vi "ComputeRelativeXYJoystickPosition.vi"(5 "Joystick Axis Info":T1, 6 "Joystick Offset":T2, 7 "reference":refnum<vi>) -> (3 "Rel XY Pos":T3)   [LabVIEW 2014]
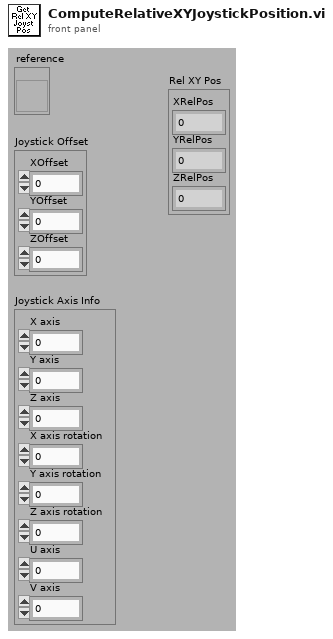
[diagram p1: front panel]
types:
  T1 = cluster{"X axis":i32, "Y axis":i32, "Z axis":i32, "X axis rotation":i32, "Y axis rotation":i32, "Z axis rotation":i32, "U axis":i32, "V axis":i32}
  T2 = cluster{"XOffset":i32, "YOffset":i32, "ZOffset":i32}
  T3 = cluster{"XRelPos":i32, "YRelPos":i32, "ZRelPos":i32}
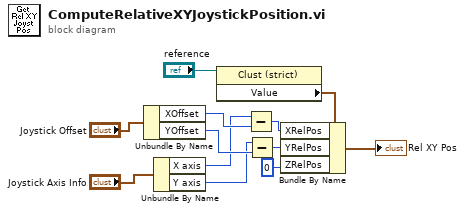
[diagram p0: block diagram]
diagram:
  n1 = Unbundle By Name("Joystick Offset") -> ("XOffset"=w8:i32, "YOffset"=w10:i32)
  n2 = Unbundle By Name("Joystick Axis Info") -> ("X axis"=w7:i32, "Y axis"=w9:i32)
  n3 = property class="Clust (strict)"(reference="reference") -> ("Value"=w11:T3)  [unwired: 1 in, 2 out]
  n4 = Subtract(x=w7, y=w8) -> (x-y=w3:i32)
  n5 = Subtract(x=w9, y=w10) -> (x-y=w4:i32)
  n6 = Bundle By Name(cluster=w11, "XRelPos"=w3, "YRelPos"=w4, "ZRelPos"=0) -> (→"Rel XY Pos":T3)
